vi "Configure Event.vi"(7 "Acquisition Number (1)":i32=1, 8 "error in (no error)":errorcluster, 9 "Repeat Count (0)":i32, 10 "Event Type (0: None)":i32(ring) items=["None", "Trigger", "Acquisition"], 11 "VISA resource name":refnum<visa-resource-name>) -> (0 "error out":errorcluster, 3 "VISA resource name out":refnum<visa-resource-name>)   [LabVIEW 2016, in "Tektronix DPO MSO 2000 4000 Series.lvlib"]
doc: "Configures the event. \n\n<B>Notes:</B>\nThis VI is available for MDO3000 Series only."
uses:
  Tektronix DPO MSO 2000 4000 Series.lvlib
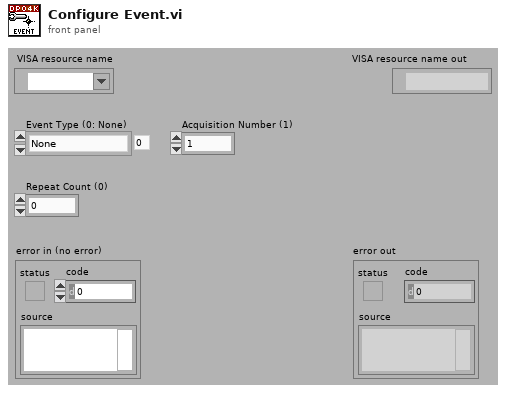
[diagram p1: front panel]
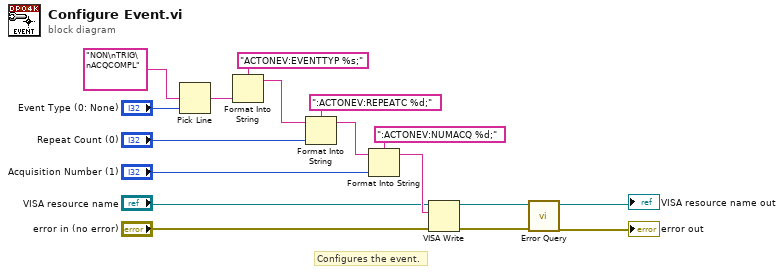
[diagram p0: block diagram]
diagram:
  # "Configures the event."
  n1 = Pick Line(multi-line string="NON\nTRIG\nACQCOMPL", line index="Event Type (0: None)") -> (output string=w3:string)  [unwired: 1 in]
  n2 = Format Into String(format string="ACTONEV:EVENTTYP %s;", w3) -> (resulting string=w16:string)  [unwired: 2 in, 1 out]
  n3 = Format Into String(format string=":ACTONEV:REPEATC %d;", initial string=w16, "Repeat Count (0)") -> (resulting string=w13:string)  [unwired: 1 in, 1 out]
  n4 = Format Into String(format string=":ACTONEV:NUMACQ %d;", initial string=w13, "Acquisition Number (1)") -> (resulting string=w10:string)  [unwired: 1 in, 1 out]
  n5 = VISA Write(VISA resource name="VISA resource name", write buffer=w10, error in (no error)="error in (no error)") -> (VISA resource name out=w8:refnum<visa-resource-name>, error out=w7:errorcluster)  [unwired: 1 out]
  n6 = call "Error Query.vi"("error in (no error)"=w7, "VISA resource name"=w8) -> ("error out"=→"error out":errorcluster, "VISA resource name out"=→"VISA resource name out":refnum<visa-resource-name>)  [unwired: 6 in, 2 out]
